vi "set_material_sensor.vi"(8 "error in (no error)":errorcluster, 9 "Sensor number":u8, 10 "Material number":u8, 11 "VISA resource name":refnum<visa-resource-name>) -> (0 "error out":errorcluster, 3 "VISA resource name out":refnum<visa-resource-name>)   [LabVIEW 2018, in "Inficon IC6.lvlib"]
doc: "Set the sensor used to measure the deposition rate of a given material."
uses:
  <instrlib>/Inficon IC6/Inficon IC6.lvlib
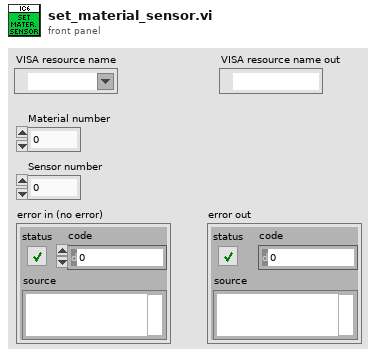
[diagram p1: front panel]
types:
  T1 = enum16{"Source", "General", "Input name", "Process name", "Logic", "Material", "Material name", "Output name", "Process", "Sensor", "Output type", "User message", "Layer", ""}
  T2 = enum16{"Hello", "Query", "Remote action", "Status", "Update"}
  T3 = cluster{"Material number":u8, "Sensor number":u8}
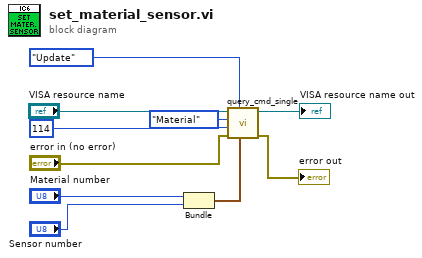
[diagram p0: block diagram]
diagram:
  n1 = Bundle("Material number"="Material number", "Sensor number"="Sensor number") -> (w6:T3)  [unwired: 1 in]
  n2 = call <instrlib>:"query_cmd_single.vi"("Parameter"=w6, "Command group"=T2."Update", "error in (no error)"="error in (no error)", "Command ID"=u8 114, "Command subgroup"=T1."Material", "VISA resource name"="VISA resource name") -> ("error out"=→"error out":errorcluster, "VISA resource name out"=→"VISA resource name out":refnum<visa-resource-name>)  [unwired: 1 in, 3 out]
